vi "Get OBJ NOT RefNum.vi"(0 "reference in":refnum<class "Generic Utilities.lvclass">, 5 "error in (no error)":errorcluster) -> (13 "OBJ not a refnum?":bool, 14 "reference out":refnum<class "Generic Utilities.lvclass">, 19 "error out":errorcluster)   [LabVIEW 2020, in "Generic Utilities.lvclass"]
uses:
  Generic Utilities.lvclass
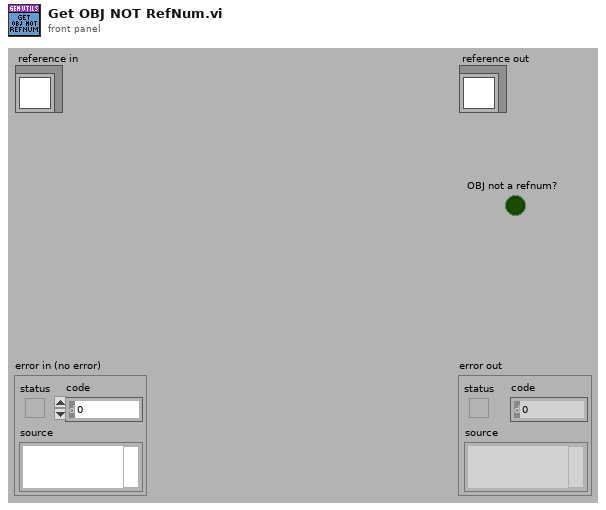
[diagram p1: front panel]
types:
  T1 = typedef "Generic Utilities.lvclass/ObjectAttributes.ctl" = cluster{"GUI Parameters":T2, "State Machine Control":cluster{"Timeout":i32, "State Queue":string[], "State History":string[], "State History Length":i32}, "Logging File Path":path, "OBJ not a refnum?":bool, "Timer Start":timestamp, "FP Refnums":T3}
  T2 = typedef "Generic Utilities.lvclass/GUI Parameters.ctl" = cluster{"Application Name":string, "GUI VI Ref":refnum<vi>, "Close Panel?":bool, "Message Window ref":refnum<vi>, "Version #":string}
  T3 = typedef "Generic Utilities.lvclass/FP Refnums.ctl" = cluster{"Panel refnum":refnum<vi>, "Control Labels":string[], "Refnums":refnum<vi>[]}
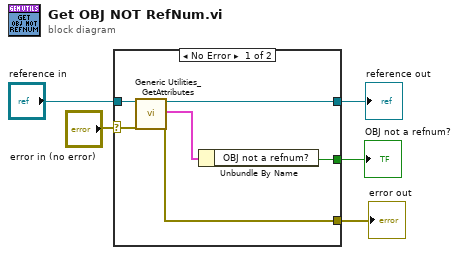
[diagram p0: block diagram]
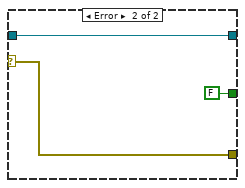
[diagram p2: hidden frame]
diagram:
  n1 = case shown="No Error" "error in (no error)" {
    selector: "error in (no error)" -> [w11 w14]
    tunnel: [w10 w14] -> w4
    tunnel: [w9 w13] -> w2
    tunnel: "reference in" -> [w7 w13]
    tunnel: [w6 FALSE ("Close Panel?")] -> w1
    frame No Error {
      n2 = call "Generic Utilities_GetAttributes.vi"("reference in"=w7, "error in (no error)"=w11) -> ("reference out"=w9:refnum<class "Generic Utilities.lvclass">, "attributes"=w8:T1, "error out"=w10:errorcluster)  [unwired: 14 in, 1 out]
      n3 = Unbundle By Name(w8) -> ("OBJ not a refnum?"=w6:bool)
    }
    frame Error {
    }
  }
  "error out" <- w4
  "reference out" <- w2
  "OBJ not a refnum?" <- w1
